vi "SeqResultHandling.vi"(8 "error in (no error)":errorcluster, 11 "TestSeqClass in":refnum<class "TestSeqClass.lvclass">) -> (0 "error out":errorcluster, 3 "TestSeqClass out":refnum<class "TestSeqClass.lvclass">)   [LabVIEW 2019, in "TestSeqClass.lvclass"]
uses:
  TestSeqClass.lvclass
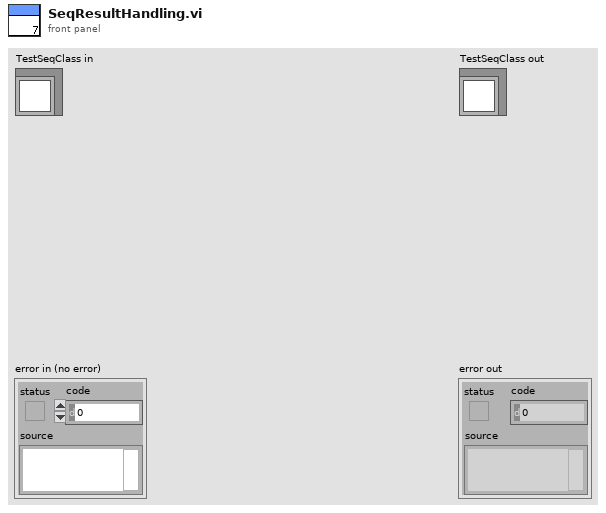
[diagram p1: front panel]
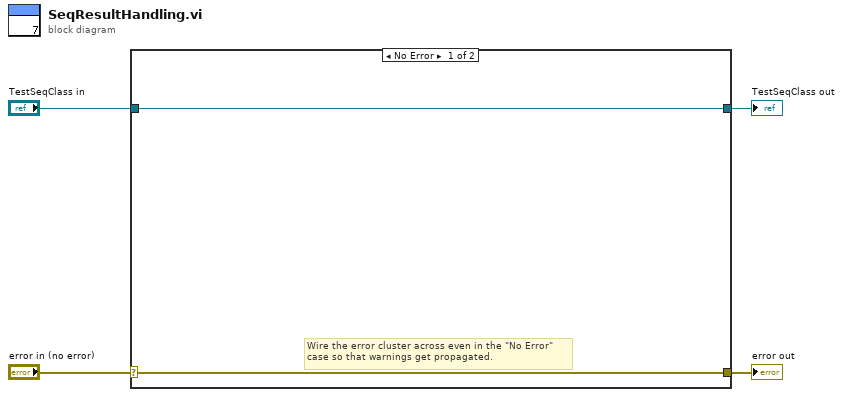
[diagram p0: block diagram]
diagram:
  n1 = case shown="No Error" "error in (no error)" {
    selector: "error in (no error)" -> [w5 w8]
    tunnel: [w5 w8] -> w3
    tunnel: [w6 w7] -> w1
    tunnel: "TestSeqClass in" -> [w6 w7]
    frame No Error {
      # "Wire the error cluster across even in the \"No Error\"\ncase so that warnings get propagated."
    }
    frame Error {
    }
  }
  "error out" <- w3
  "TestSeqClass out" <- w1
